vi "change_password.vi"() -> ()   [LabVIEW 2013, in "main.lvlib"]
uses:
  main.lvlib
panel:
  in  "Cancel":bool
  in  "PresentPassword":string caption="Nuværende Kodeord"
  in  "RetypePassword":string caption="Gentag"
  in  "Submit":bool
  in  "NewPassword":string caption="Nyt Kodeord"
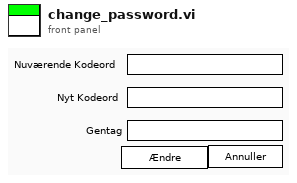
[diagram p1: front panel]
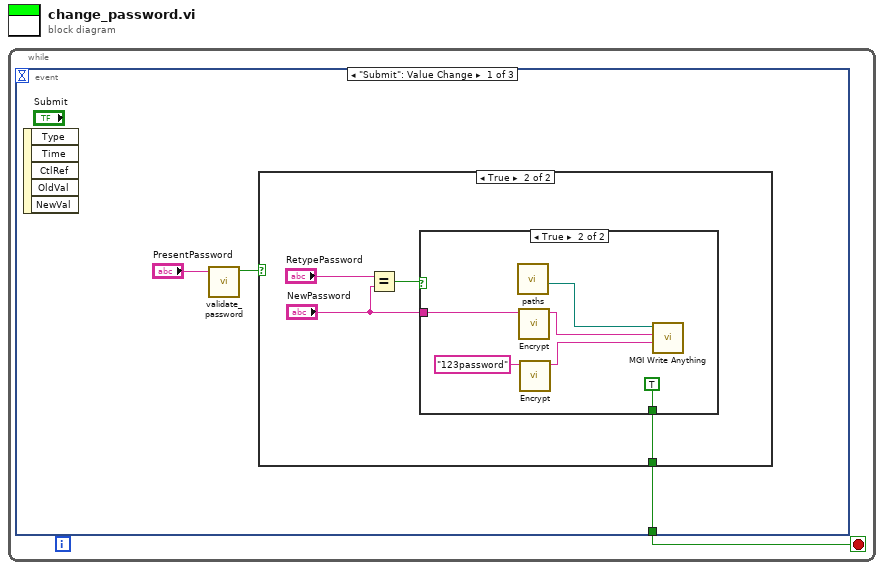
[diagram p0: block diagram]
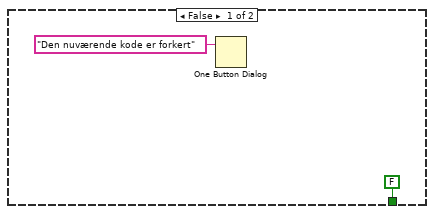
[diagram p2: hidden frame]
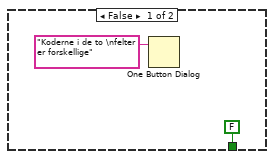
[diagram p3: hidden frame]
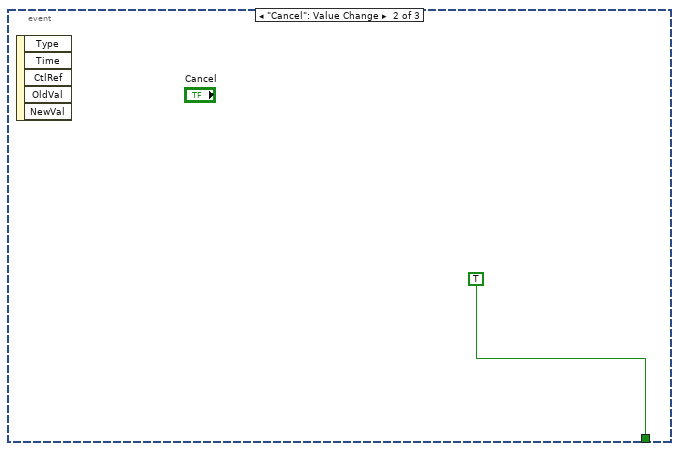
[diagram p4: hidden frame]
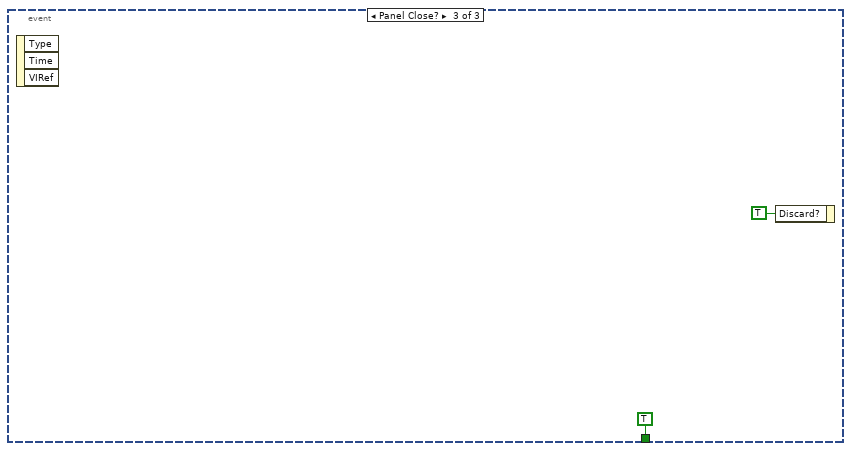
[diagram p5: hidden frame]
diagram:
  n1 = while {
    stop <- w1 stop-if-true
    n2 = event shown="[0] \"Submit\": Value Change" {
      selector: _ -> [_ _ _]
      dyn-events: _ -> [_ _ _]
      timeout: _ -> [_ _ _]
      tunnel: [w4 TRUE TRUE] -> w1
      event "Submit": Value Change {
        n3 = event-data() -> ()  [unwired: 1 in, 5 out]
        n4 = call "validate_password.vi"("Password"="PresentPassword") -> ("Accept"=w2:bool)  [unwired: 10 in]
        n5 = case shown="True" w2 {
          tunnel: [FALSE w7] -> w4
          frame False {
            n6 = One Button Dialog(message="Den nuværende kode er forkert") -> ()  [unwired: 1 in, 1 out]
          }
          frame True {
            n7 = Equal?(x="RetypePassword", y="NewPassword") -> (x = y?=w8:bool)
            n8 = case shown="True" w8 {
              tunnel: "NewPassword" -> [_ w14]
              tunnel: [FALSE TRUE] -> w7
              frame False {
                n9 = One Button Dialog(message="Koderne i de to \nfelter er forskellige") -> ()  [unwired: 1 in, 1 out]
              }
              frame True {
                n10 = call "paths.vi"() -> ("Controlsettings2"=w15:path)  [unwired: 8 in, 3 out]
                n11 = call "Encrypt.vi"("Input"=w14) -> ("Output"=w16:string)  [unwired: 10 in]
                n12 = call "Encrypt.vi"("Input"="123password") -> ("Output"=w17:string)  [unwired: 10 in]
                n13 = call <userlib>:"MGI Write Anything.vi"("Section Name (Name of \"Anything\")"=w17, "Anything"=w16, "Path (dialog)"=w15) -> ()  [unwired: 6 in, 3 out]
              }
            }
          }
        }
      }
      event "Cancel": Value Change {
        n14 = event-data() -> ()  [unwired: 1 in, 5 out]
      }
      event Panel Close? {
        n15 = event-data() -> ()  [unwired: 1 in, 3 out]
        n16 = event-data("Discard?"=TRUE) -> ()  [unwired: 1 in, 1 out]
      }
    }
  }
